vi "Demo Power Electronics--constant.vi"() -> (3 "Nombre":string="Francisco")   [LabVIEW 2024, in "Cloneable.lvlib"]
uses:
  Cloneable.lvlib
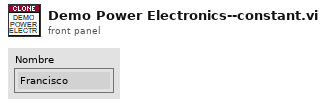
[diagram p1: front panel]
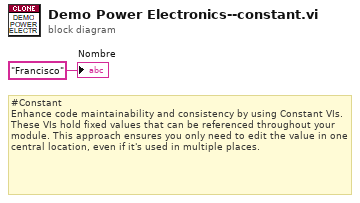
[diagram p0: block diagram]
diagram:
  # "#Constant\nEnhance code maintainability and consistency by using Constant VIs. These VIs hold fixed values that can be referenced throughout your module. This approach ensures you only need to edit the value in one central location, even if it's used in multiple places."
  "Nombre" <- "Francisco" ("Nombre")
